vi "sv_Convert Value to String (Direction).vi"(7 "direction value":T1 items=["-Z Rotation"=-6, "-Y Rotation"=-5, "-X Rotation"=-4, "-Z Translation"=-3, "-Y Translation"=-2, "-X Translation"=-1, "Scalar"=0, "+X Translation"=1, "+Y Translation"=2, "+Z Translation"=3, "+X Rotation"=4, "+Y Rotation"=5, "+Z Rotation"=6]) -> (8 "direction string":string)   [LabVIEW 2017, in "SoundVib_UFF58.lvlib"]
uses:
  <vilib>/addons/Sound and Vibration/svt_UFF58/SoundVib_UFF58.lvlib
  <vilib>/addons/Sound and Vibration/svt_UFF58/subVIs/sv_UFF58 Response Direction.ctl
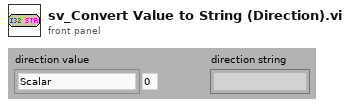
[diagram p1: front panel]
types:
  T1 = typedef "SoundVib_UFF58.lvlib/sv_UFF58 Response Direction.ctl" = i32
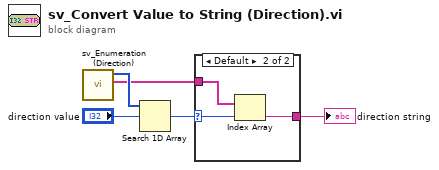
[diagram p0: block diagram]
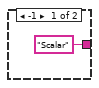
[diagram p2: hidden frame]
diagram:
  n1 = call <vilib>:"sv_Enumeration (Direction).vi"() -> ("direction strings"=w3:string[], "direction values"=w4:T1[])  [unwired: 10 in]
  n2 = Search 1D Array(1D array=w4, element="direction value") -> (index of element=w5:i32)  [unwired: 1 in]
  n3 = case shown="Default" w5 {
    selector: w5 -> [_ w8]
    tunnel: ["Scalar" w7] -> w1
    tunnel: w3 -> [_ w9]
    frame -1 {
    }
    frame Default {
      n4 = Index Array(array=w9, index=w8) -> (element=w7:string)
    }
  }
  "direction string" <- w1
